vi "sensor por.vi"() -> ()   [LabVIEW 2016]
uses:
  <vilib>/LabVIEW Interface for Arduino/Type Defs/Board Type.ctl
  <vilib>/LabVIEW Interface for Arduino/Type Defs/Connection Type.ctl
  <vilib>/LabVIEW Interface for Arduino/Type Defs/Pin Mode.ctl
  <vilib>/LabVIEW Interface for Arduino/LabVIEW Interface for Arduino.lvlib
panel:
  in  "stop":bool
  out "Boolean":bool
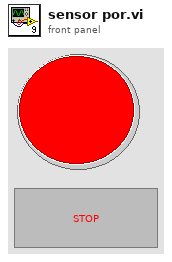
[diagram p1: front panel]
types:
  T1 = typedef "LabVIEW Interface for Arduino.lvlib/Pin Mode.ctl" = enum8{"Input", "Output"}
  T2 = typedef "LabVIEW Interface for Arduino.lvlib/Connection Type.ctl" = enum8{"USB / Serial", "XBEE", "BlueSmirf (Bluetooth)"}
  T3 = typedef "LabVIEW Interface for Arduino.lvlib/Board Type.ctl" = enum16{"Uno", "Dimuelanove w/Atmega 328", "Mega 2560"}
  T4 = typedef "LabVIEW Interface for Arduino.lvlib/Arduino Resource.ctl" = cluster{"VISA resource":refnum<visa-resource-name>, "Board Type":T3, "Connection Type":enum8{"USB / Serial"}, "Bytes Per Packet (15)":u8}
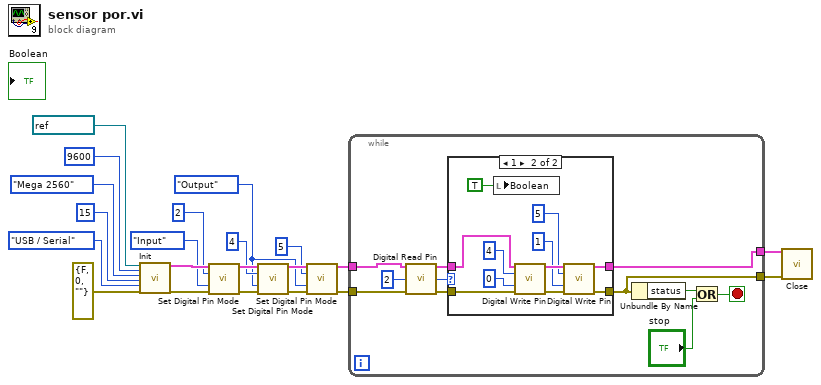
[diagram p0: block diagram]
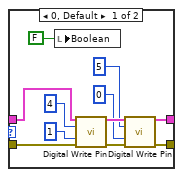
[diagram p2: hidden frame]
diagram:
  w5 = Pin_Mode."Output" ("Pin Mode (Input)")
  n1 = call <vilib>:"Init.vi"("VISA resource"=refnum<visa-resource-name> "COM6", "Baud Rate (115200)"=u32 9600, "Board Type (Uno)"=Board_Type."Mega 2560", "Bytes Per Packet (15)"=u32 15, "Connection Type (USB/Serial)"=Connection_Type."USB / Serial", "error in"=errorcluster {"status"=FALSE, "code"=0, "source"=""}) -> ("Arduino Resource"=w11:T4, "error out"=w10:errorcluster)  [unwired: 12 in]
  n2 = call <vilib>:"Set Digital Pin Mode.vi"("Arduino Resource"=w11, "Digital I/O Pin"=u8 2, "Pin Mode (Input)"=Pin_Mode."Input", "error in"=w10) -> ("Arduino Resource"=w15:T4, "error out"=w14:errorcluster)  [unwired: 10 in]
  n3 = call <vilib>:"Set Digital Pin Mode.vi"("Arduino Resource"=w15, "Digital I/O Pin"=u8 4, "Pin Mode (Input)"=w5, "error in"=w14) -> ("Arduino Resource"=w13:T4, "error out"=w12:errorcluster)  [unwired: 10 in]
  n4 = call <vilib>:"Set Digital Pin Mode.vi"("Arduino Resource"=w13, "Digital I/O Pin"=u8 5, "Pin Mode (Input)"=w5, "error in"=w12) -> ("Arduino Resource"=w4:T4, "error out"=w3:errorcluster)  [unwired: 10 in]
  n5 = while {
    tunnel: w4 -> [w31]
    tunnel: w3 -> [w30]
    tunnel: [w26] -> w2
    tunnel: [w22] -> w1
    stop <- w25 stop-if-true
    n6 = call <vilib>:"Digital Read Pin.vi"("Arduino Resource"=w31, "Digital I/O Pin (0)"=u8 2, "error in"=w30) -> ("Arduino Resource"=w28:T4, "Value"=w29:u8, "error out"=w27:errorcluster)  [unwired: 10 in]
    n7 = case shown="1" w29 {
      tunnel: w28 -> [w34 w54]
      tunnel: w27 -> [w33 w53]
      tunnel: [w36 w45] -> w26
      tunnel: [w35 w44] -> w22
      frame 0, Default {
        n8 = local write "Boolean"(FALSE ("Boolean")) -> ()
        n9 = call <vilib>:"Digital Write Pin.vi"("Arduino Resource"=w34, "Digital I/O Pin (0)"=u8 4, "Value (0)"=u8 1, "error in"=w33) -> ("Arduino Resource"=w42:T4, "error out"=w43:errorcluster)  [unwired: 10 in]
        n10 = call <vilib>:"Digital Write Pin.vi"("Arduino Resource"=w42, "Digital I/O Pin (0)"=u8 5, "Value (0)"=u8 0, "error in"=w43) -> ("Arduino Resource"=w36:T4, "error out"=w35:errorcluster)  [unwired: 10 in]
      }
      frame 1 {
        n11 = local write "Boolean"(TRUE ("Boolean")) -> ()
        n12 = call <vilib>:"Digital Write Pin.vi"("Arduino Resource"=w54, "Digital I/O Pin (0)"=u8 4, "Value (0)"=u8 0, "error in"=w53) -> ("Arduino Resource"=w51:T4, "error out"=w52:errorcluster)  [unwired: 10 in]
        n13 = call <vilib>:"Digital Write Pin.vi"("Arduino Resource"=w51, "Digital I/O Pin (0)"=u8 5, "Value (0)"=u8 1, "error in"=w52) -> ("Arduino Resource"=w45:T4, "error out"=w44:errorcluster)  [unwired: 10 in]
      }
    }
    n14 = Unbundle By Name(w22) -> ("status"=w24:bool)
    n15 = Or(x=w24, y="stop") -> (x .or. y?=w25:bool)
  }
  n16 = call <vilib>:"Close.vi"("Arduino Resource"=w2, "error in"=w1) -> ()  [unwired: 13 in, 1 out]
